vi "Differential_delay_line_configuration_Mezzaninev56.vi"() -> ()   [LabVIEW 2009]
panel:
  out "connection ID out":refnum<k5>
  in  "connection ID in":refnum<k5>
  out "Delay value 2":u16(ring) items=["0", "0.25ns", "0.5ns", "0.75ns", "1ns", "1.25ns", "1.5ns", "1.75ns", "2ns", "2.25ns", "2.5ns", "2.75ns", "3ns", "3.25ns", "3.5ns", "3.75ns", "4ns", "4.25ns", "4.5ns", "4.75ns", "5ns", "5.25ns", "5.5ns", "5.75ns", "2ns_b", "2.25ns_b", "2.5ns_b", "2.75ns_b", "3ns_b", "3.25ns_b", "3.5ns_b", "3.75ns_b", ""]
  in  "Delay value":u16(ring) items=["0ns", "0.25ns", "0.5ns", "0.75ns", "1ns", "1.25ns", "1.5ns", "1.75ns", "2ns", "2.25ns", "2.5ns", "2.75ns", "3ns", "3.25ns", "3.5ns", "3.75ns", "4ns", "4.25ns", "4.5ns", "4.75ns", "5ns", "5.25ns", "5.5ns", "5.75ns", "2ns_b", "2.25ns_b", "2.5ns_b", "2.75ns_b", "3ns_b", "3.25ns_b", "3.5ns_b", "3.75ns_b"]
  in  "channel":i32
  out "data read value 18":u32
  out "Value hex":u32
  out "Data to send hex 18":string
  out "data out serial 18":string
  in  "Id in":i32
  out "Id out":i32
  out "error out":errorcluster
  in  "error in (no error)":errorcluster
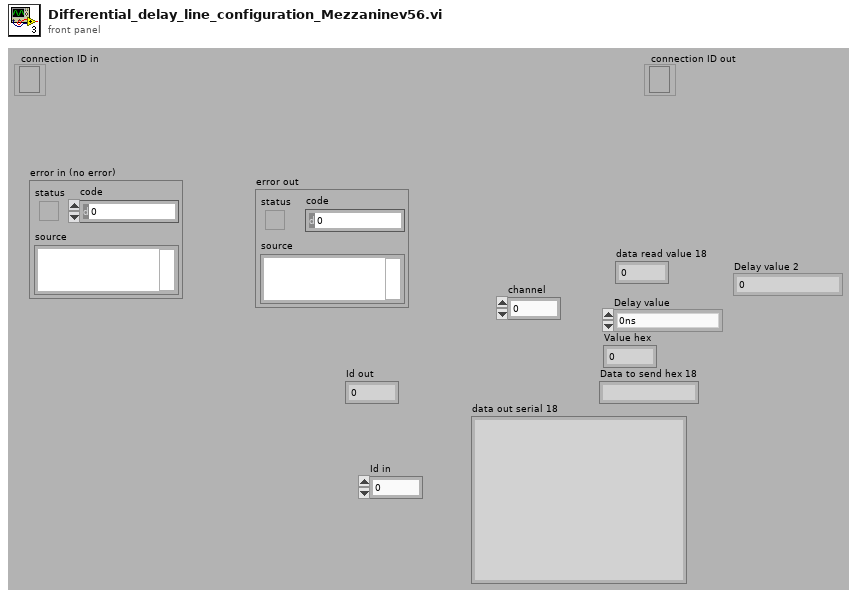
[diagram p1: front panel]
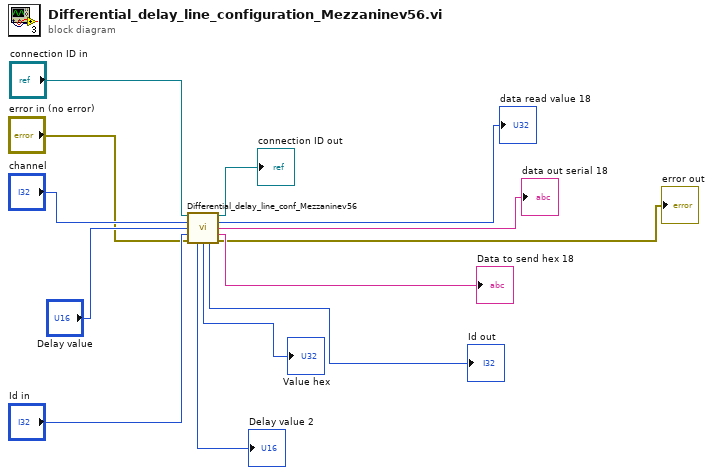
[diagram p0: block diagram]
diagram:
  n1 = call "Differential_delay_line_conf_Mezzaninev56.vi"("connection ID out"="connection ID in", "channel"="channel", "Delay value"="Delay value", "Id in"="Id in", "error out 2"="error in (no error)") -> ("connection ID out 2"=→"connection ID out":refnum<k5>, "data read value 18"=→"data read value 18":u32, "data out serial 18"=→"data out serial 18":string, "Data to send hex 18"=→"Data to send hex 18":string, "Delay value 2"=→"Delay value 2":u16, "Value hex"=→"Value hex":u32, "Id out"=→"Id out":i32, "error out 3"=→"error out":errorcluster)  [unwired: 3 in]
